vi "ExFileReadNDisplay.vi"() -> ()   [LabVIEW 2010]
panel:
  in  "Full File Name":path
  in  "?":bool
  in  "FileType":u32=67371008
  out "error out":errorcluster
  in  "error in (no error)":errorcluster
  # "ExReadFileNDisplay.vi\nThis example will read in a file of the\nselected data type and display all frames.\nWhen finished viewing data, make sure to\nuse the STOP button to close the display."
  # "File Types:\nSPE = 67371008\nTIF   = 67174400\nPMI  = 67436544"
  # "Browse match pattern is set to *.tif.  Modify this if different file type is needed."
  # "NOTICE\n\nTHIS VI REQUIRES THAT THE TOOLKIT\nBE UNLOADED BY RUNNING THE\n VI EXCLOSEGLOBALCAM.VI\n BEFORE LEAVING LABVIEW."
  # "This will properly close\nthe image and\ndeallocate memory."
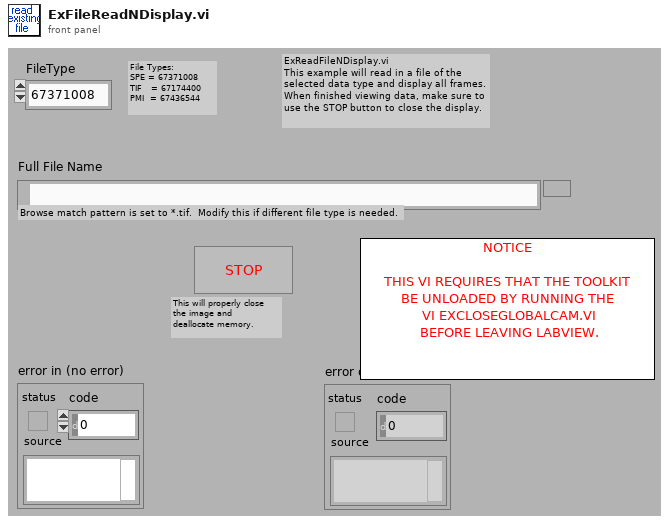
[diagram p1: front panel]
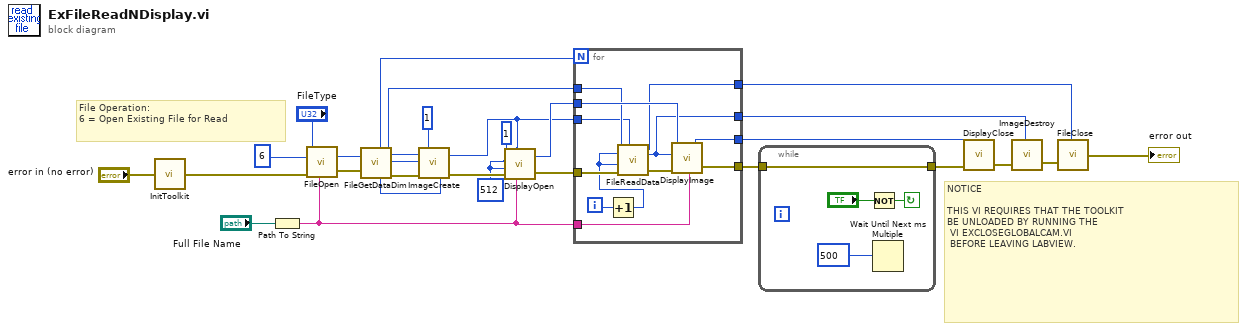
[diagram p0: block diagram]
diagram:
  w16 = 512
  # "NOTICE\n\nTHIS VI REQUIRES THAT THE TOOLKIT\nBE UNLOADED BY RUNNING THE\n VI EXCLOSEGLOBALCAM.VI\n BEFORE LEAVING LABVIEW."
  # "File Operation:\n6 = Open Existing File for Read"
  n1 = call <userlib>:"InitToolkit.vi"("error in"="error in (no error)") -> ("error out"=w27:errorcluster)
  n2 = Path To String(path="Full File Name") -> (string=w2:string)
  n3 = call <userlib>:"FileOpen.vi"("error in"=w27, "File Operations"=u32 6 ("File Operation"), "FileName"=w2, "File Type"="FileType") -> ("error out"=w25:errorcluster, "File Handle"=w24:u32)
  n4 = call <userlib>:"FileGetDataDim.vi"("File Handle"=w24, "error in"=w25) -> ("Number of Frames"=w18:u32, "Data Type"=w20:u32, "File Handle"=w12:u32, "X dim"=w22:u32, "Y dim"=w21:u32, "error out"=w23:errorcluster)
  n5 = call <userlib>:"ImageCreate.vi"("X dimension"=w22, "Y dimension"=w21, "Data Type"=w20, "error in"=w23, "Number Of Frames"=1) -> ("Image Handle"=w11:u32, "error out"=w19:errorcluster)
  n6 = call <userlib>:"DisplayOpen.vi"("Display Title"=w2, "Image Handle"=w11, "error in"=w19, "Display Height"=w16, "Display Width"=w16, "Display Type"=1) -> ("error out"=w14:errorcluster, "Display Handle"=w13:u32)
  n7 = for {
    N: w18 -> [_]
    tunnel: w14 -> [w41]
    tunnel: w13 -> [w39]
    tunnel: w12 -> [w38]
    tunnel: w11 -> [w37]
    tunnel: [w34] -> w4
    tunnel: [w33] -> w10
    tunnel: [w32] -> w9
    tunnel: [w31] -> w6
    tunnel: w2 -> [w30]
    i -> [w36]
    n8 = Increment(x=w36) -> (x+1=w35:i32)
    n9 = call <userlib>:"FileReadData.vi"("File Handle"=w38, "Start Frame"=w35, "End Frame"=w35, "error in"=w41, "Image Handle"=w37) -> ("File Handle"=w32:u32, "Image Handle"=w31:u32, "error out"=w40:errorcluster)
    n10 = call <userlib>:"DisplayImage.vi"("error in"=w40, "Title"=w30, "Image Handle"=w31, "Display Handle"=w39) -> ("error out"=w34:errorcluster, "Display Handle"=w33:u32)
  }
  n11 = while {
    tunnel: w4 -> [w45]
    tunnel: [w45] -> w5
    stop <- w43 continue-if-true
    n12 = Not(x="?") -> (.not. x?=w43:bool)
    n13 = Wait Until Next ms Multiple(millisecond multiple=500) -> ()  [unwired: 1 out]
  }
  n14 = call <userlib>:"DisplayClose.vi"("error in"=w5, "Display Handle"=w10) -> ("error out"=w8:errorcluster)
  n15 = call <userlib>:"ImageDestroy.vi"("error in"=w8, "Data handle"=w6) -> ("error out"=w7:errorcluster)
  n16 = call <userlib>:"FileClose.vi"("error in"=w7, "File Handle"=w9) -> ("error out"=→"error out":errorcluster)
